vi "Pulse and Transition Measurements.vi"() -> ()   [LabVIEW 2020]
doc: "This example shows the use of cursors to display the results of certain waveform measurement calculations within a graph."
uses:
  <vilib>/measure/mascope.llb/Transition Measurements 1 chan.vi
  <vilib>/measure/mascope.llb/Pulse Measurements.vi
  <vilib>/measure/mascope.llb/Cycle Average and RMS.vi
  <vilib>/measure/mascope.llb/Amplitude and Levels.vi
  <vilib>/Waveform/WDTOps.llb/WDT Get Final Time Value DBL.vi
  <vilib>/measure/NI_MAPro.lvlib
  <vilib>/measure/NI_MABase.lvlib
panel:
  in  "Measurements":u16(ring) items=["Transition", "Pulse", "Cycle Average and RMS", "Amplitude and Level"]
  in  "Zoom?":bool
  out "Simulated Data":waveform(dbl)(graph)
  in  "Stop":bool
  # "Overview: Demonstrates the use of cursors to display the results of certain waveform measurement calculations within a graph.\nRequirements: LabVIEW Full Development System\nInstructions:\n1. Run the VI.\n2. Change the value of the Measurements ring to see cursors displayed for a particular type of measurement.\n3. Click the Zoom? button to zoom the graph display on the applicable area of the graph.\n4. Click Stop to stop the VI."
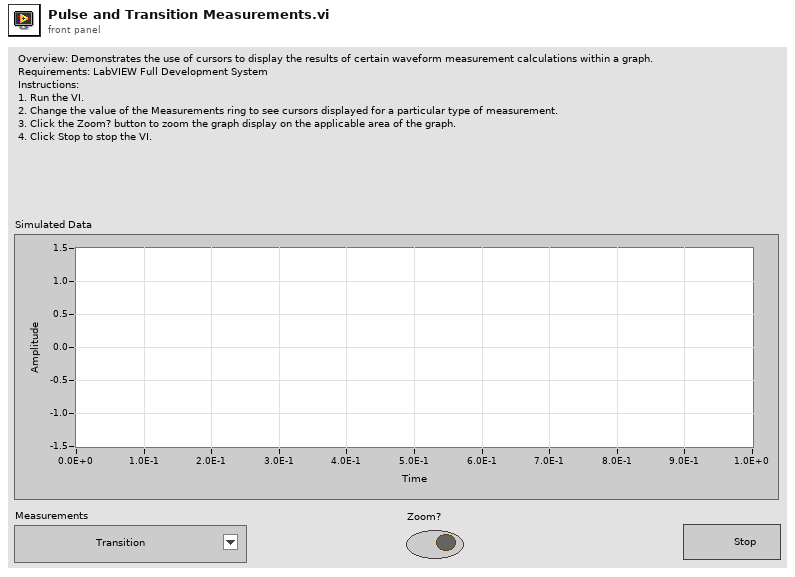
[diagram p1: front panel]
types:
  T1 = enum16{"Sine Wave", "Triangle Wave", "Square Wave", "Sawtooth Wave"}
  T2 = cluster{"method":enum32{"histogram", "peak", "auto select"}, "histogram size":i32, "histogram method":enum16{"mode"}, "reserved":dbl}
  T3 = cluster{"high ref level":dbl, "mid ref level":dbl, "low ref level":dbl, "ref units":u16}
  T4 = cluster{"start time":dbl, "end time":dbl, "ref levels":cluster{"high ref level":dbl, "mid ref level":dbl, "low ref level":dbl, "ref units":u16}}
  T5 = cluster{"pulse center":dbl, "ref levels":cluster{"high ref level":dbl, "mid ref level":dbl, "low ref level":dbl, "ref units":u16}}
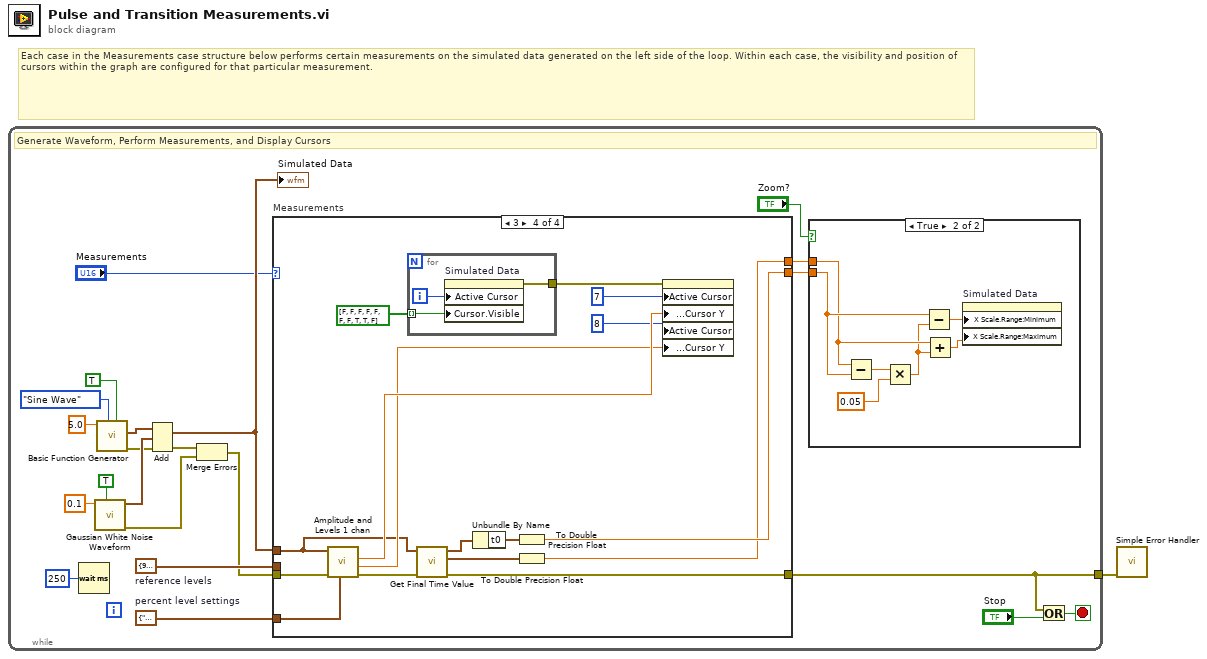
[diagram p0: block diagram]
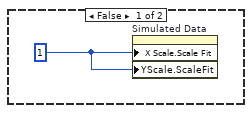
[diagram p2: hidden frame]
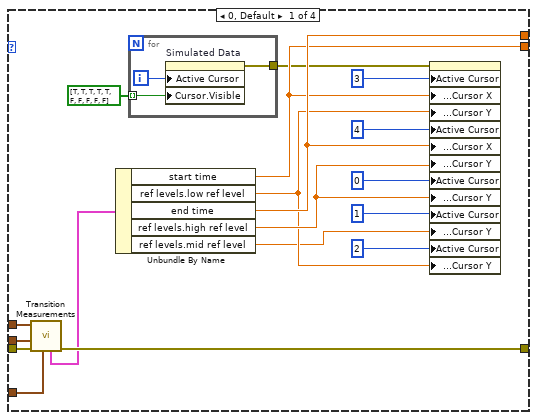
[diagram p3: hidden frame]
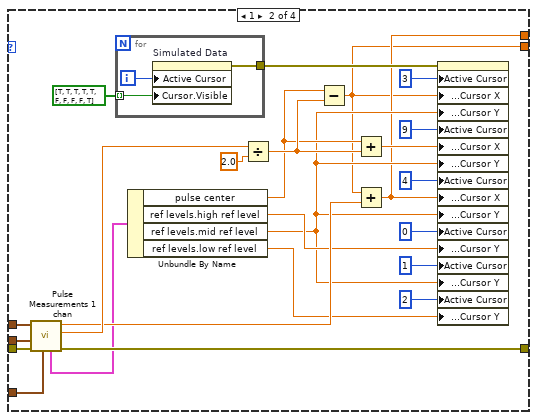
[diagram p4: hidden frame]
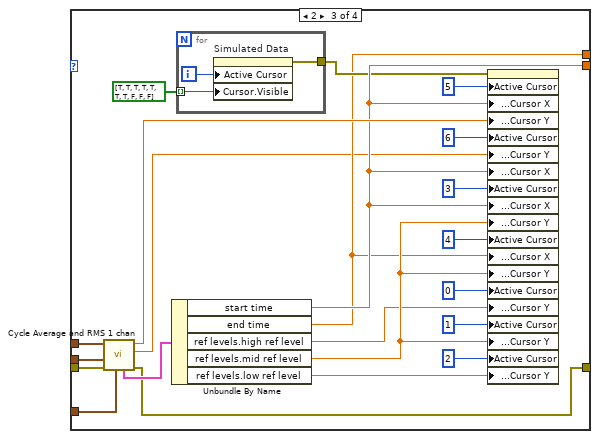
[diagram p5: hidden frame]
diagram:
  # "Each case in the Measurements case structure below performs certain measurements on the simulated data generated on the left side of the loop. Within each case, the visibility and position of cursors within the graph are configured for that particular measurement."
  n1 = while {
    tunnel: [w10] -> w1
    stop <- w14 stop-if-true
    w20 = T2 {"method"=enum."auto select", "histogram size"=256, "histogram method"=enum."mode", "reserved"=1.0}  # percent level settings
    w19 = T3 {"high ref level"=90.0, "mid ref level"=50.0, "low ref level"=10.0, "ref units"=1}  # reference levels
    # "Generate Waveform, Perform Measurements, and Display Cursors"
    n2 = Wait (ms)(milliseconds to wait=u32 250) -> ()  [unwired: 1 out]
    n3 = call <vilib>:"Gaussian White Noise Waveform.vi"("reset signal"=TRUE, "standard deviation"=0.1 ("noise std dev")) -> ("error out"=w5:errorcluster, "signal out"=w12:waveform(dbl))  [unwired: 8 in]
    n4 = call <vilib>:"Basic Function Generator.vi"("reset signal"=TRUE, "signal type"=T1."Sine Wave", "frequency"=5.0) -> ("error out"=w7:errorcluster, "signal out"=w13:waveform(dbl))  [unwired: 6 in, 1 out]
    n5 = Add(1:w12, 2:w13, 4:w7) -> (0:w18:waveform(dbl), 3:w6:errorcluster)
    "Simulated Data" <- w18
    n6 = Merge Errors(w6, w5) -> (w4:errorcluster)
    n7 = case "Measurements" shown="3" "Measurements" {
      tunnel: w18 -> [w49 w77 w102 w116]
      tunnel: w20 -> [w47 w75 w100 w121]
      tunnel: w19 -> [w48 w76 w101 _]
      tunnel: [w40 w59 w97 w118] -> w17
      tunnel: [w43 w60 w89 w112] -> w16
      tunnel: [w46 w68 w95 w108] -> w10
      tunnel: w4 -> [w45 w67 w94 w114]
      frame 0, Default {
        n8 = call-poly <vilib>:"Transition Measurements.vi"("percent level settings"=w47, "error in (no error)"=w45, "reference levels"=w48, "signal in"=w49) -> ("error out"=w46:errorcluster, "measurement info"=w37:T4)  [unwired: 2 in, 4 out]
        n9 = Unbundle By Name(w37) -> ("start time"=w40:dbl, "ref levels.low ref level"=w42:dbl, "end time"=w43:dbl, "ref levels.high ref level"=w44:dbl, "ref levels.mid ref level"=w41:dbl)
        n10 = for {
          tunnel: [w51] -> w39
          tunnel: bool[] [TRUE, TRUE, TRUE, TRUE, TRUE, FALSE, FALSE, FALSE, FALSE, FALSE] -> [w50] mode=indexing
          i -> [w52]
          n11 = property on="Simulated Data" class="WFGraph (strict)"("Active Cursor"=w52, "Cursor.Visible"=w50) -> (error out=w51:errorcluster)  [unwired: 2 in, 1 out]
        }
        n12 = property on="Simulated Data" class="WFGraph (strict)"(error in=w39, "Active Cursor"=u32 3, "Cursor.Cursor Position:Cursor X"=w40, "Cursor.Cursor Position:Cursor Y"=w42, "Active Cursor"=u32 4, "Cursor.Cursor Position:Cursor X"=w43, "Cursor.Cursor Position:Cursor Y"=w44, "Active Cursor"=u32 0, "Cursor.Cursor Position:Cursor Y"=w44, "Active Cursor"=u32 1, "Cursor.Cursor Position:Cursor Y"=w41, "Active Cursor"=u32 2, "Cursor.Cursor Position:Cursor Y"=w42) -> ()  [unwired: 1 in, 2 out]
      }
      frame 1 {
        n13 = call-poly <vilib>:"Pulse Measurements 1 chan.vi"("percent level settings"=w75, "error in (no error)"=w67, "reference levels"=w76, "signal in"=w77) -> ("error out"=w68:errorcluster, "pulse duration"=w74:dbl, "period"=w73:dbl, "measurement info"=w64:T5)  [unwired: 3 in, 1 out]
        n14 = for {
          tunnel: [w79] -> w66
          tunnel: bool[] [TRUE, TRUE, TRUE, TRUE, TRUE, FALSE, FALSE, FALSE, FALSE, TRUE] -> [w78] mode=indexing
          i -> [w80]
          n15 = property on="Simulated Data" class="WFGraph (strict)"("Active Cursor"=w80, "Cursor.Visible"=w78) -> (error out=w79:errorcluster)  [unwired: 2 in, 1 out]
        }
        n16 = Unbundle By Name(w64) -> ("pulse center"=w71:dbl, "ref levels.high ref level"=w69:dbl, "ref levels.mid ref level"=w61:dbl, "ref levels.low ref level"=w62:dbl)
        n17 = Divide(x=w74, y=2.0) -> (x/y=w72:dbl)
        n18 = Subtract(x=w71, y=w72) -> (x-y=w59:dbl)
        n19 = Add(x=w71, y=w72) -> (x+y=w70:dbl)
        n20 = Add(x=w59, y=w73) -> (x+y=w60:dbl)
        n21 = property on="Simulated Data" class="WFGraph (strict)"(error in=w66, "Active Cursor"=u32 3, "Cursor.Cursor Position:Cursor X"=w59, "Cursor.Cursor Position:Cursor Y"=w61, "Active Cursor"=u32 9, "Cursor.Cursor Position:Cursor X"=w70, "Cursor.Cursor Position:Cursor Y"=w61, "Active Cursor"=u32 4, "Cursor.Cursor Position:Cursor X"=w60, "Cursor.Cursor Position:Cursor Y"=w61, "Active Cursor"=u32 0, "Cursor.Cursor Position:Cursor Y"=w69, "Active Cursor"=u32 1, "Cursor.Cursor Position:Cursor Y"=w61, "Active Cursor"=u32 2, "Cursor.Cursor Position:Cursor Y"=w62) -> ()  [unwired: 1 in, 2 out]
      }
      frame 2 {
        n22 = call-poly <vilib>:"Cycle Average and RMS 1 chan.vi"("percent level settings"=w100, "error in (no error)"=w94, "reference levels"=w101, "signal in"=w102) -> ("error out"=w95:errorcluster, "cycle RMS"=w88:dbl, "cycle average"=w99:dbl, "measurement info"=w98:T4)  [unwired: 4 in]
        n23 = Unbundle By Name(w98) -> ("start time"=w97:dbl, "end time"=w89:dbl, "ref levels.high ref level"=w90:dbl, "ref levels.mid ref level"=w91:dbl, "ref levels.low ref level"=w96:dbl)
        n24 = for {
          tunnel: [w104] -> w93
          tunnel: bool[] [TRUE, TRUE, TRUE, TRUE, TRUE, TRUE, TRUE, FALSE, FALSE, FALSE] -> [w103] mode=indexing
          i -> [w105]
          n25 = property on="Simulated Data" class="WFGraph (strict)"("Active Cursor"=w105, "Cursor.Visible"=w103) -> (error out=w104:errorcluster)  [unwired: 2 in, 1 out]
        }
        n26 = property on="Simulated Data" class="WFGraph (strict)"(error in=w93, "Active Cursor"=u32 5, "Cursor.Cursor Position:Cursor X"=w97, "Cursor.Cursor Position:Cursor Y"=w99, "Active Cursor"=u32 6, "Cursor.Cursor Position:Cursor Y"=w88, "Cursor.Cursor Position:Cursor X"=w97, "Active Cursor"=u32 3, "Cursor.Cursor Position:Cursor X"=w97, "Cursor.Cursor Position:Cursor Y"=w91, "Active Cursor"=u32 4, "Cursor.Cursor Position:Cursor X"=w89, "Cursor.Cursor Position:Cursor Y"=w91, "Active Cursor"=u32 0, "Cursor.Cursor Position:Cursor Y"=w90, "Active Cursor"=u32 1, "Cursor.Cursor Position:Cursor Y"=w91, "Active Cursor"=u32 2, "Cursor.Cursor Position:Cursor Y"=w96) -> ()  [unwired: 1 in, 2 out]
      }
      frame 3 {
        n27 = call-poly <vilib>:"Amplitude and Levels 1 chan.vi"("state settings"=w121, "error in (no error)"=w114, "signal in"=w116) -> ("error out"=w109:errorcluster, "low state level"=w119:dbl, "high state level"=w120:dbl)  [unwired: 5 in, 1 out]
        n28 = for {
          tunnel: [w123] -> w111
          tunnel: bool[] [FALSE, FALSE, FALSE, FALSE, FALSE, FALSE, FALSE, TRUE, TRUE, FALSE] -> [w122] mode=indexing
          i -> [w124]
          n29 = property on="Simulated Data" class="WFGraph (strict)"("Active Cursor"=w124, "Cursor.Visible"=w122) -> (error out=w123:errorcluster)  [unwired: 2 in, 1 out]
        }
        n30 = call-poly <vilib>:"Get Final Time Value.vi"("error in (no error)"=w109, "waveform in"=w116) -> ("error out"=w108:errorcluster, "tf"=w117:timestamp, "waveform out"=w115:waveform(dbl))  [unwired: 7 in]
        n31 = Unbundle By Name(w115) -> ("t0"=w113:timestamp)
        n32 = To Double Precision Float(number=w113) -> (double precision float=w118:dbl)
        n33 = To Double Precision Float(number=w117) -> (double precision float=w112:dbl)
        n34 = property on="Simulated Data" class="WFGraph (strict)"(error in=w111, "Active Cursor"=u32 7, "Cursor.Cursor Position:Cursor Y"=w120, "Active Cursor"=u32 8, "Cursor.Cursor Position:Cursor Y"=w119) -> ()  [unwired: 1 in, 2 out]
      }
    }
    n35 = case shown="True" "Zoom?" {
      tunnel: w17 -> [_ w30]
      tunnel: w16 -> [_ w29]
      frame False {
        w24 = u8 1
        n36 = property on="Simulated Data" class="WFGraph (strict)"("X Scale.Scale Fit"=w24, "YScale.ScaleFit"=w24) -> ()  [unwired: 2 in, 2 out]
      }
      frame True {
        n37 = Subtract(x=w29, y=w30) -> (x-y=w31:dbl)
        n38 = Multiply(x=w31, y=0.05) -> (x*y=w28:dbl)
        n39 = Subtract(x=w30, y=w28) -> (x-y=w27:dbl)
        n40 = Add(x=w29, y=w28) -> (x+y=w26:dbl)
        n41 = property on="Simulated Data" class="WFGraph (strict)"("X Scale.Range:Minimum"=w27, "X Scale.Range:Maximum"=w26) -> ()  [unwired: 2 in, 2 out]
      }
    }
    n42 = Or(x=w10, y="Stop") -> (x .or. y?=w14:bool)
  }
  n43 = call <vilib>:"Simple Error Handler.vi"("error in (no error)"=w1) -> ()  [unwired: 4 in, 5 out]
